vi "Decorations Loop.vi"(8 "error in (no error)":errorcluster, 9 "Decos[]":refnum<vi>[](array[refnum]), 11 "Material-Scheme in":refnum<class "Material-Scheme.lvclass">) -> (0 "error out":errorcluster)   [LabVIEW 2026, in "TSC Material Theme.lvlib" / "Material-Scheme.lvclass"]
doc: "Change the coloring on decorations\n-> If it is a text decoration, change the background color only when it wasn't transparent before AND change the text color; otherwise, normal decoration just change background/foreground\n\n<b>Code Developed By:</b> +\nDaniel Coons +\nTechnology Service Corporation +\nwww.tsc.com/atcs"
uses:
  Material-Scheme.lvclass
  Material-Scheme.lvclass/Material-Scheme.ctl
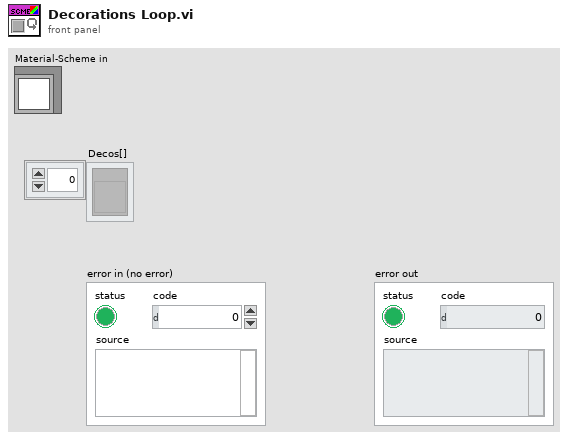
[diagram p1: front panel]
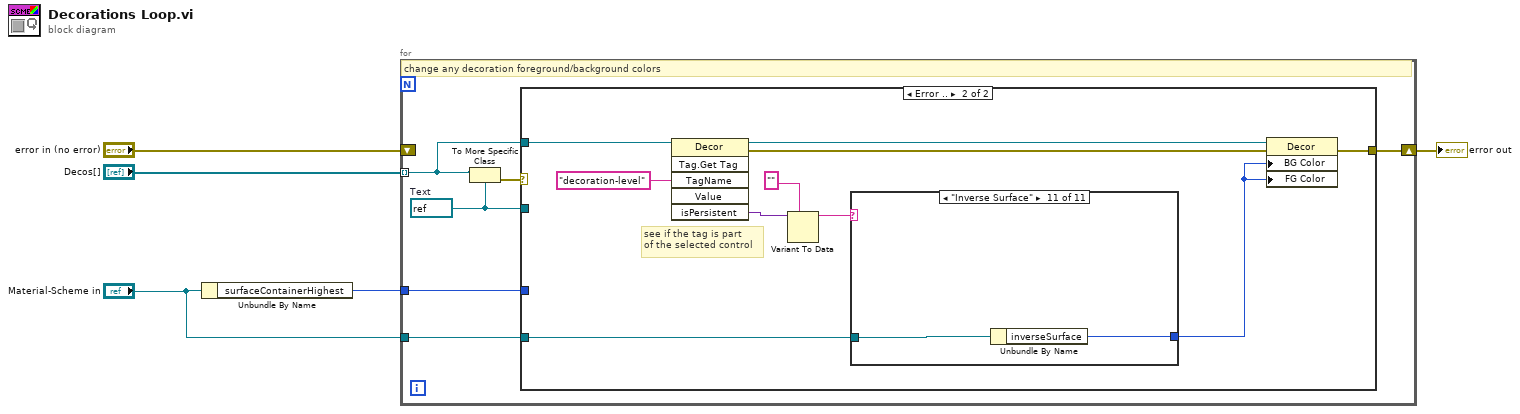
[diagram p0: block diagram]
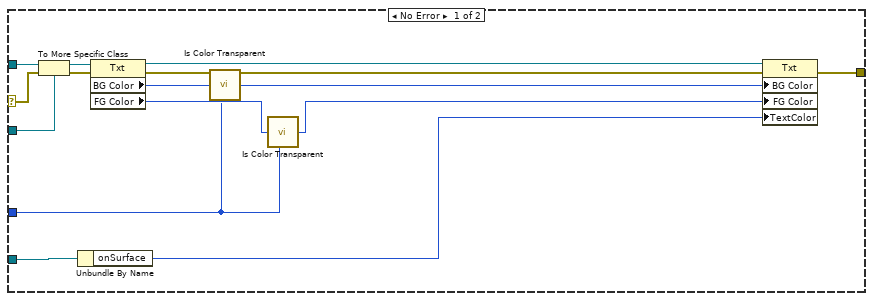
[diagram p2: hidden frame]
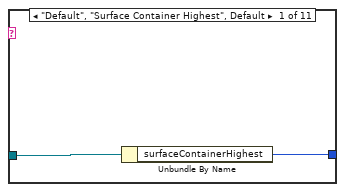
[diagram p3: hidden frame]
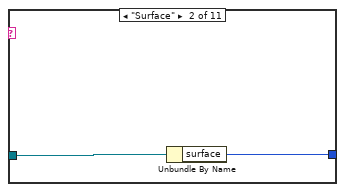
[diagram p4: hidden frame]
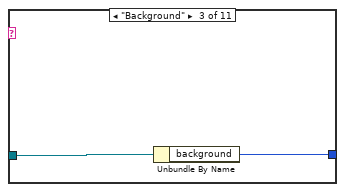
[diagram p5: hidden frame]
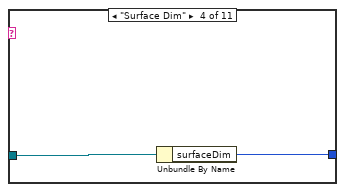
[diagram p6: hidden frame]
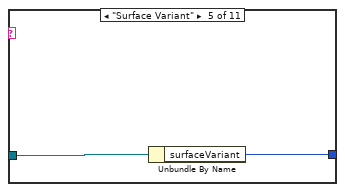
[diagram p7: hidden frame]
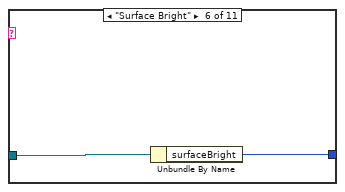
[diagram p8: hidden frame]
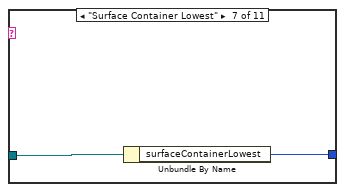
[diagram p9: hidden frame]
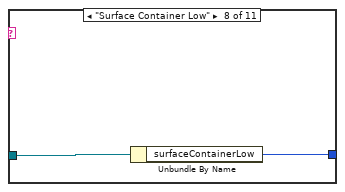
[diagram p10: hidden frame]
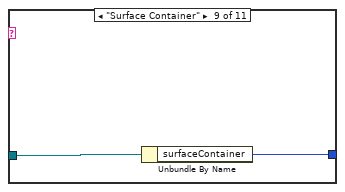
[diagram p11: hidden frame]
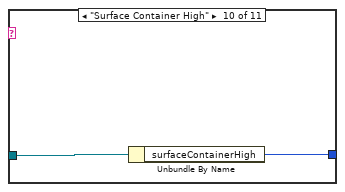
[diagram p12: hidden frame]
diagram:
  n1 = Unbundle By Name("Material-Scheme in") -> ("surfaceContainerHighest"=w2:u32)
  n2 = for {
    shift-right: [w11] -> w3
    shift-left: "error in (no error)" -> [_]
    tunnel: "Decos[]" -> [w8] mode=indexing
    tunnel: w2 -> [w10]
    tunnel: "Material-Scheme in" -> [w6]
    w7 = refnum<vi> refnum  # Text
    # "change any decoration foreground/background colors"
    n3 = To More Specific Class(target class=w7, reference=w8) -> (error out=w9:errorcluster)  [unwired: 1 in, 1 out]
    n4 = case shown="Error .." w9 {
      selector: w9 -> [w25 _]
      tunnel: [w26 w36] -> w11
      tunnel: w10 -> [w14 _]
      tunnel: w8 -> [w23 w32]
      tunnel: w7 -> [w24 _]
      tunnel: w6 -> [w13 w31]
      frame No Error {
        n5 = To More Specific Class(target class=w24, reference=w23, error in=w25) -> (specific class reference=w20:refnum<vi>, error out=w22:errorcluster)
        n6 = Unbundle By Name(w13) -> ("onSurface"=w12:u32)
        n7 = property class="Txt"(reference=w20, error in=w22) -> (reference out=w19:refnum<vi>, error out=w21:errorcluster, "BG Color"=w18:u32, "FG Color"=w16:u32)
        n8 = call "Is Color Transparent.vi"("original color"=w18, "desired color"=w14) -> ("updated color"=w17:u32)  [unwired: 3 in]
        n9 = call "Is Color Transparent.vi"("original color"=w16, "desired color"=w14) -> ("updated color"=w15:u32)  [unwired: 3 in]
        n10 = property class="Txt"(reference=w19, error in=w21, "BG Color"=w17, "FG Color"=w15, "TextColor"=w12) -> (error out=w26:errorcluster)  [unwired: 1 out]
      }
      frame Error {
        # "see if the tag is part \nof the selected control"
        n11 = invoke class="Decor" method="Tag.Get Tag"(reference=w32, "TagName"="decoration-level" ("Tag Name")) -> (reference out=w28:refnum<vi>, error out=w27:errorcluster, "isPersistent"=w34:variant)  [unwired: 4 in, 3 out]
        n12 = Variant To Data(type="", Variant=w34) -> (data=w30:string)  [unwired: 1 in, 1 out]
        n13 = case shown="\"Inverse Surface\"" w30 {
          tunnel: w31 -> [w38 w40 w42 w44 w46 w48 w50 w52 w54 w56 w58]
          tunnel: [w37 w39 w41 w43 w45 w47 w49 w51 w53 w55 w57] -> w29
          frame "Default", "Surface Container Highest", Default {
            n14 = Unbundle By Name(w38) -> ("surfaceContainerHighest"=w37:u32)
          }
          frame "Surface" {
            n15 = Unbundle By Name(w40) -> ("surface"=w39:u32)
          }
          frame "Background" {
            n16 = Unbundle By Name(w42) -> ("background"=w41:u32)
          }
          frame "Surface Dim" {
            n17 = Unbundle By Name(w44) -> ("surfaceDim"=w43:u32)
          }
          frame "Surface Variant" {
            n18 = Unbundle By Name(w46) -> ("surfaceVariant"=w45:u32)
          }
          frame "Surface Bright" {
            n19 = Unbundle By Name(w48) -> ("surfaceBright"=w47:u32)
          }
          frame "Surface Container Lowest" {
            n20 = Unbundle By Name(w50) -> ("surfaceContainerLowest"=w49:u32)
          }
          frame "Surface Container Low" {
            n21 = Unbundle By Name(w52) -> ("surfaceContainerLow"=w51:u32)
          }
          frame "Surface Container" {
            n22 = Unbundle By Name(w54) -> ("surfaceContainer"=w53:u32)
          }
          frame "Surface Container High" {
            n23 = Unbundle By Name(w56) -> ("surfaceContainerHigh"=w55:u32)
          }
          frame "Inverse Surface" {
            n24 = Unbundle By Name(w58) -> ("inverseSurface"=w57:u32)
          }
        }
        n25 = property class="Decor"(reference=w28, error in=w27, "BG Color"=w29, "FG Color"=w29) -> (error out=w36:errorcluster)  [unwired: 1 out]
      }
    }
  }
  "error out" <- w3
